vi "lv Add Arr.vi"(8 "error in (no error)":errorcluster) -> (0 "error out":errorcluster)   [LabVIEW 2020, in "1DVectorDll.lvlib"]
doc: "_declspec(dllexport) void lvAddArr(TD1Hd1 arr0, TD1Hd1 arr1);"
uses:
  1DVectorDll.lvlib
  1DVectorDll.dll
panel:
  out "arr1 2":dbl[](array[numeric])=[1.0, 2.0, 3.0, 5.0, 7.0, 8.0]
  out "arr0 2":dbl[](array[numeric])=[1.0, 0.0, 4.0, 5.0]
  in  "arr1":dbl[](array[numeric])=[1.0, 2.0, 3.0, 5.0, 7.0, 8.0]
  in  "arr0":dbl[](array[numeric])=[0.0, 0.0, 4.0, 5.0]
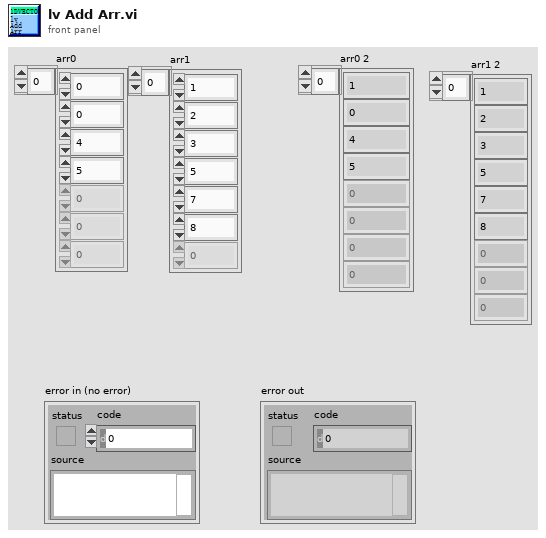
[diagram p1: front panel]
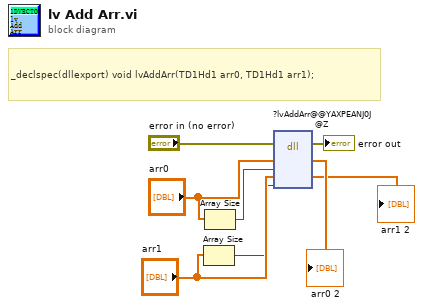
[diagram p0: block diagram]
diagram:
  # "_declspec(dllexport) void lvAddArr(TD1Hd1 arr0, TD1Hd1 arr1);"
  n1 = Array Size(array="arr1") -> (size(s)=w1:i32)
  n2 = Array Size(array="arr0") -> (size(s)=w3:i32)
  n3 = dll-call lib="E:/Practice/Lv/dll/CppDllForLv/src/1DVectorDll/lv/1DVectorDll.*" fn="?lvAddArr@@YAXPEANJ0J@Z"(error in="error in (no error)", "arr0"="arr0", "size0"=w3, "arr1"="arr1", "size1"=w1) -> (error out=→"error out":errorcluster, "arr0"=→"arr0 2":dbl[], "arr1"=→"arr1 2":dbl[])  [unwired: 5 in, 1 out]
